vi "make_dc_array (SubVI).vi"(11 "DC supply settings:":T1) -> (3 "Tot DC Arr":dbl[][](array[numeric]))   [LabVIEW 2014]
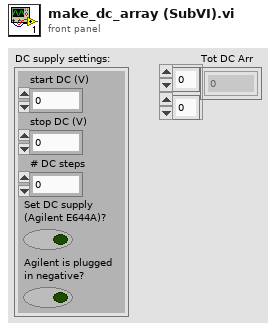
[diagram p1: front panel]
types:
  T1 = cluster{"start DC (V)":ext, "stop DC (V)":ext, "# DC steps ":i32, "Set DC supply\n(Agilent E644A)? ":bool, "Agilent is plugged \nin negative?":bool}
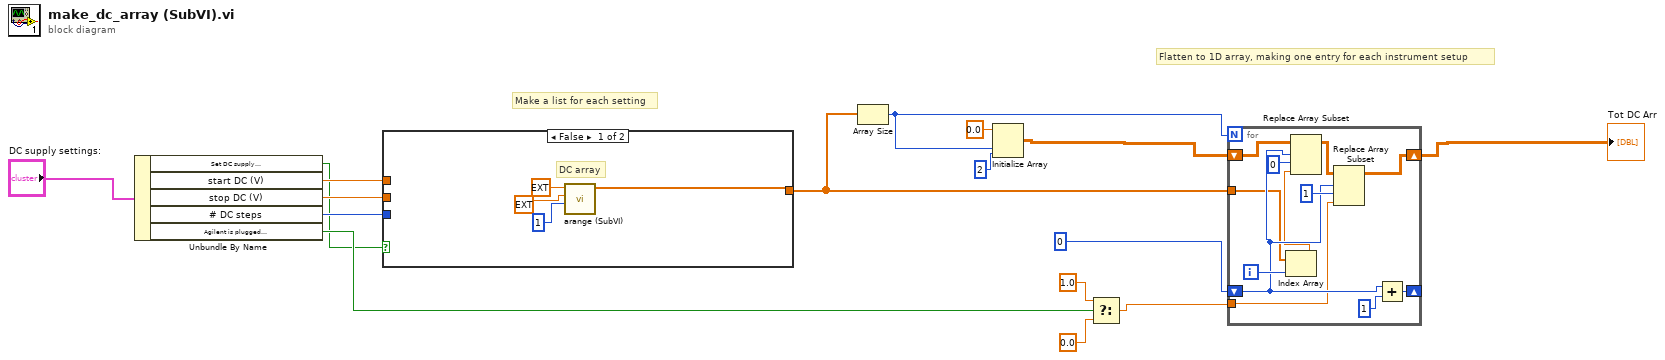
[diagram p0: block diagram]
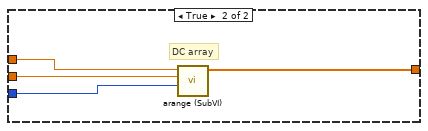
[diagram p2: hidden frame]
diagram:
  # "Make a list for each setting"
  # "Flatten to 1D array, making one entry for each instrument setup"
  n1 = Unbundle By Name("DC supply settings:") -> ("Set DC supply\n(Agilent E644A)?"=w1:bool, "start DC (V)"=w2:ext, "stop DC (V)"=w3:ext, "# DC steps"=w4:i32, "Agilent is plugged \nin negative?"=w13:bool)
  n2 = case shown="False" w1 {
    tunnel: w2 -> [_ w24]
    tunnel: w3 -> [_ w23]
    tunnel: w4 -> [_ w22]
    tunnel: [w17 w21] -> w12
    frame False {
      # "DC array"
      n3 = call "arange (SubVI).vi"("# Steps"=1, "stop"=ext -1.0, "start"=ext -1.0) -> ("Array"=w17:ext[])  [unwired: 8 in]
    }
    frame True {
      # "DC array"
      n4 = call "arange (SubVI).vi"("# Steps"=w22, "stop"=w23, "start"=w24) -> ("Array"=w21:ext[])  [unwired: 8 in]
    }
  }
  n5 = Array Size(array=w12) -> (size(s)=w11:i32)
  n6 = Initialize Array(0.0 ("element"), w11, 2 ("dimension size")) -> (w7:dbl[][])
  n7 = Select(t=1.0, s=w13, f=0.0) -> (s? t:f=w16:dbl)
  n8 = for {
    N: w11 -> [_]
    shift-right: [w28] -> w9
    shift-left: w7 -> [w36]
    shift-right: [w30] -> _
    shift-left: 0 ("disabled index (row)") -> [w29]
    tunnel: w12 -> [w27]
    tunnel: w16 -> [w25]
    i -> [w32]
    n9 = Index Array(array=w27, index=w32) -> (element=w26:ext)
    n10 = Replace Array Subset(array=w36, new element=w26, index (row)=w29, index (col)=0 ("disabled index (col)")) -> (w34:dbl[][])
    n11 = Replace Array Subset(array=w34, new element=w25, index (row)=w29, index (col)=1 ("disabled index (col)")) -> (w28:dbl[][])
    n12 = Add(x=w29, y=1) -> (x+y=w30:i32)
  }
  "Tot DC Arr" <- w9
